vi "Lowpass Filter.vi"(1 "Ts [s]":dbl=0.1 min=0.0, 2 "Tf [s]":dbl=2.0 min=0.0, 3 "Filter Input":dbl=20.0) -> (0 "Filter Output":dbl=20.0)   [LabVIEW 2018]
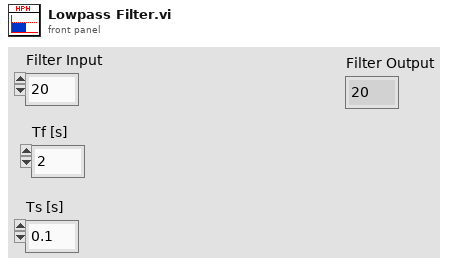
[diagram p1: front panel]
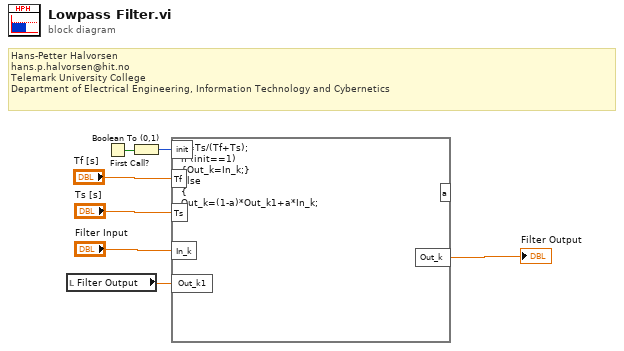
[diagram p0: block diagram]
diagram:
  # "Hans-Petter Halvorsen\nhans.p.halvorsen@hit.no\nTelemark University College \nDepartment of Electrical Engineering, Information Technology and Cybernetics"
  n1 = local read "Filter Output"() -> (w3:dbl)
  n2 = First Call?() -> (First Call?: T/F=w1:bool)
  n3 = Boolean To (0,1)(Boolean=w1) -> (0, 1=w2:i16)
  n4 = formula code="a=Ts/(Tf+Ts);\nif (init==1)\n{Out_k=In_k;}\nelse\n{\nOut_k=(1-a)*Out_k1+a*In_k;\n}"("Tf"="Tf [s]", "Ts"="Ts [s]", "Out_k1"=w3, "In_k"="Filter Input", "init"=w2) -> ("Out_k"=→"Filter Output":dbl)  [unwired: 1 out]
